vi "Daxsonics Read Write_2.vi"(7 "Enable Termination\nChar (T)":bool=TRUE, 10 "write buffer":string, 11 "VISA resource name":refnum<visa-resource-name>="ASRL4::INSTR") -> (0 "error out":errorcluster, 2 "read buffer":string)   [LabVIEW 2022 SP3]
uses:
  <vilib>/Instr/_visa.llb/VISA Configure Serial Port (Instr).vi
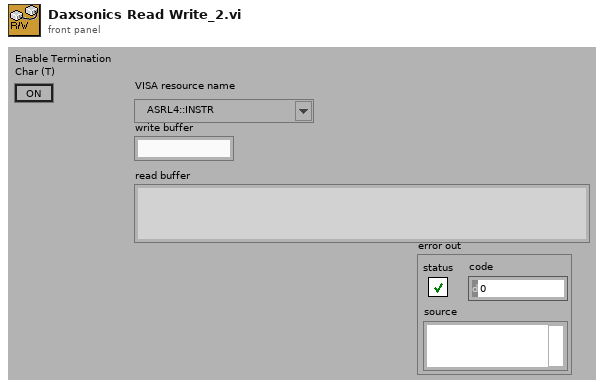
[diagram p1: front panel]
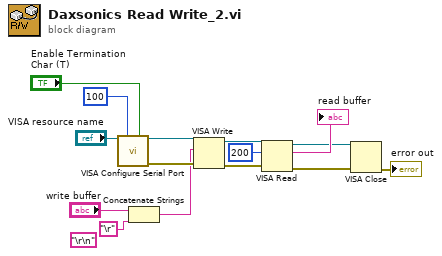
[diagram p0: block diagram]
diagram:
  (unwired) "\r\n"
  n1 = call-poly "VISA Configure Serial Port"("VISA resource name"="VISA resource name", "timeout (10sec)"=u32 100, "Enable Termination\nChar (T)"="Enable Termination\nChar (T)") -> ("VISA resource name out"=w15:refnum<visa-resource-name>, "error out"=w14:errorcluster)  [unwired: 11 in]
  n2 = Concatenate Strings("write buffer", "\r") -> (w5:string)
  n3 = VISA Write(VISA resource name=w15, write buffer=w5, error in (no error)=w14) -> (VISA resource name out=w12:refnum<visa-resource-name>, error out=w11:errorcluster)  [unwired: 1 out]
  n4 = VISA Read(VISA resource name=w12, byte count=u32 200, error in (no error)=w11) -> (VISA resource name out=w8:refnum<visa-resource-name>, read buffer=→"read buffer":string, error out=w7:errorcluster)  [unwired: 1 out]
  n5 = VISA Close(VISA resource name=w8, error in (no error)=w7) -> (error out=→"error out":errorcluster)
